vi "SLSC Convert EDS Property to Tree Control Item.vi"(6 "Enum string":cluster{"name":string, "enum":string}[](array[cluster]), 11 "property":T1) -> (2 "Glyph":i32, 3 "Child Text":string[](array[string]))   [LabVIEW 2017, in "SLSC Tree Control.lvlib"]
doc: "Convert the EDS property datatype to a Tree Control Child Text."
uses:
  SLSC Tree Control.lvlib
  Ctrl/Property.ctl
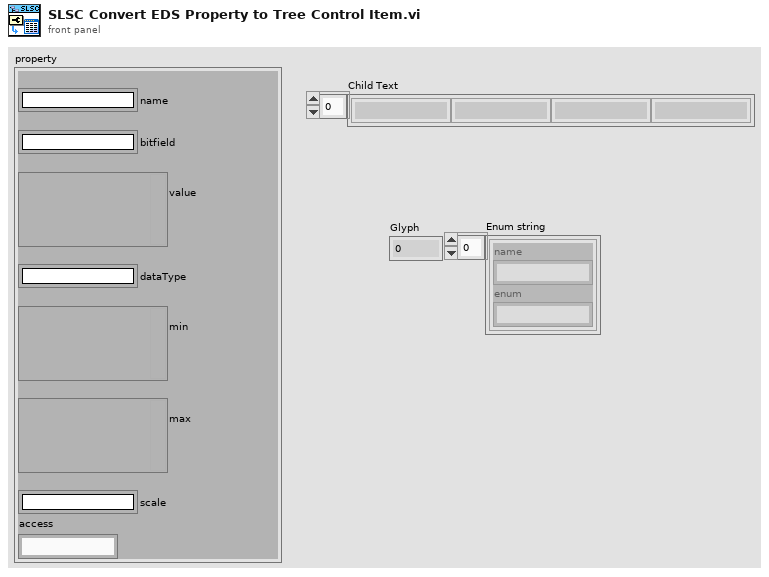
[diagram p1: front panel]
types:
  T1 = typedef "Property.ctl" = cluster{"name":string, "bitfield":string, "value":variant, "dataType":string, "min":variant, "max":variant, "scale":string, "access":string}
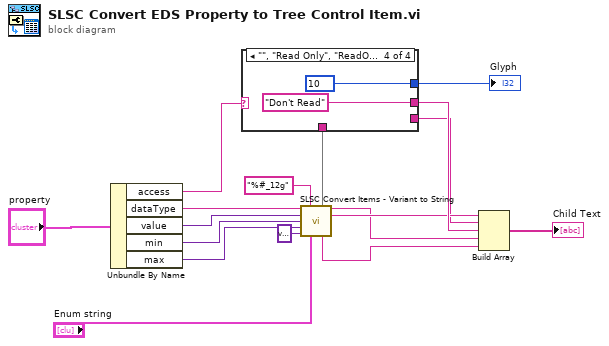
[diagram p0: block diagram]
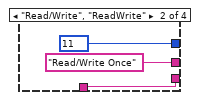
[diagram p3: hidden frame]
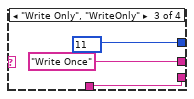
[diagram p4: hidden frame]
diagram:
  n1 = Unbundle By Name("property") -> ("access"=w11:string, "dataType"=w15:string, "value"=w14:variant, "min"=w13:variant, "max"=w9:variant)
  n2 = call "SLSC Convert Items - Variant to String.vi"("dataType"=w15, "format string"="%#_12g", "value"=w14, "min"=w13, "max"=w9, 11:variant ("reset value"), "string enums"="Enum string") -> (3:w3, "Output data type"=w4:string, "string offline data value"=w5:string, "data_range"=w6:string)  [unwired: 3 in, 2 out]
  n3 = case shown="\"\", \"Read Only\", \"ReadOnly\"" w11 {
    tunnel: [_ "Read/Write Once" ("string") "Write Once" ("string") "Don't Read" ("string")] -> w10
    tunnel: [_ 11 11 10] -> w12
    tunnel: [_ w18 w21 _] -> w2
    tunnel: w3 -> [_ w18 w21 _]
    frame Default {
    }
    frame "Read/Write", "ReadWrite" {
    }
    frame "Write Only", "WriteOnly" {
    }
    frame "", "Read Only", "ReadOnly" {
    }
  }
  "Glyph" <- w12
  n4 = Build Array(w5, w2, w10, w4, w6) -> (→"Child Text":string[])
